vi "init.vi"(8 "error in (no error)":errorcluster, 10 "Init Data":variant, 11 "Pressure Monitor in":refnum<class "Pressure Monitor.lvclass">) -> (0 "error out":errorcluster, 2 "Channel List":refnum<class "HK Item.lvclass">[](array[class]), 3 "Pressure Monitor out":refnum<class "Pressure Monitor.lvclass">)   [LabVIEW 2024, in "Pressure Monitor.lvclass"]
uses:
  Pressure Monitor.lvclass
  hk-channel-class/hk-channel-class/HK Item/HK Item.lvclass
  Pressure Monitor.lvclass/Pressure Monitor.ctl
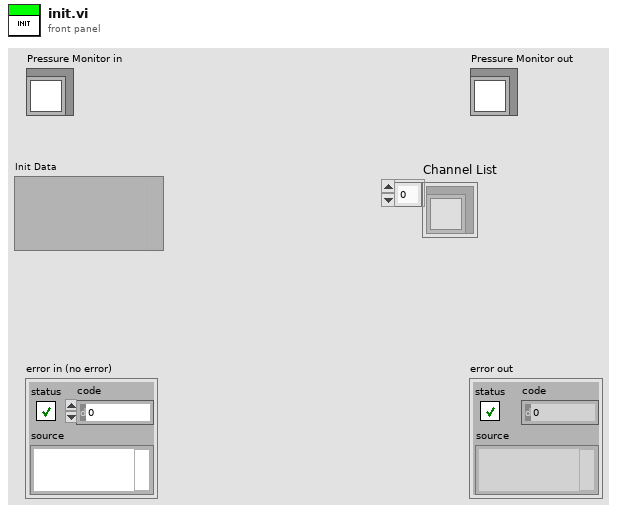
[diagram p1: front panel]
types:
  T1 = typedef "Pressure Monitor.lvclass/Pressure Settings.ctl" = cluster{"Pressure Alarm Level":dbl}
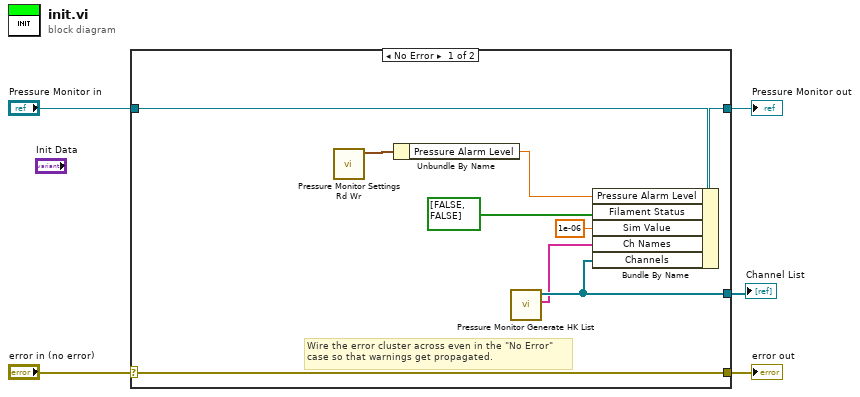
[diagram p0: block diagram]
diagram:
  n1 = case shown="No Error" "error in (no error)" {
    selector: "error in (no error)" -> [w14 w16]
    tunnel: [w14 w16] -> w4
    tunnel: [w12 w15] -> w2
    tunnel: "Pressure Monitor in" -> [w11 w15]
    tunnel: [w13 _] -> w1
    frame No Error {
      # "Wire the error cluster across even in the \"No Error\"\ncase so that warnings get propagated."
      n2 = call "Pressure Monitor Settings Rd Wr.vi"() -> ("Pressure Settings"=w7:T1)  [unwired: 10 in, 1 out]
      n3 = Unbundle By Name(w7) -> ("Pressure Alarm Level"=w6:dbl)
      n4 = call "Pressure Monitor Generate HK List.vi"() -> ("Channel Names"=w10:string[], "Channel List"=w13:refnum<class "HK Item.lvclass">[])  [unwired: 10 in]
      n5 = Bundle By Name(cluster=w11, "Pressure Alarm Level"=w6, "Filament Status"=bool[] [FALSE, FALSE], "Sim Value"=1e-06, "Ch Names"=w10, "Channels"=w13) -> (w12:refnum<class "Pressure Monitor.lvclass">)
    }
    frame Error {
    }
  }
  "error out" <- w4
  "Pressure Monitor out" <- w2
  "Channel List" <- w1
